vi "waitingStop.vi"(2 "error in (no error)":errorcluster, 3 "UART in":refnum<visa-resource-name>) -> (0 "error out":errorcluster, 1 "UART out":refnum<visa-resource-name>)   [LabVIEW 2016]
panel:
  out "String":string
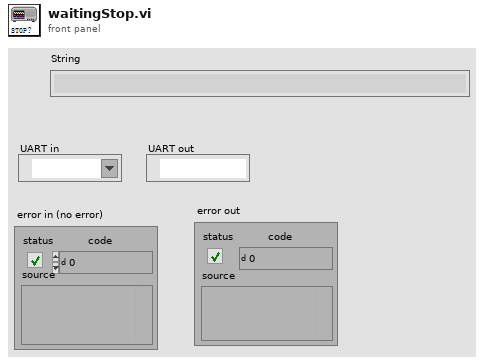
[diagram p1: front panel]
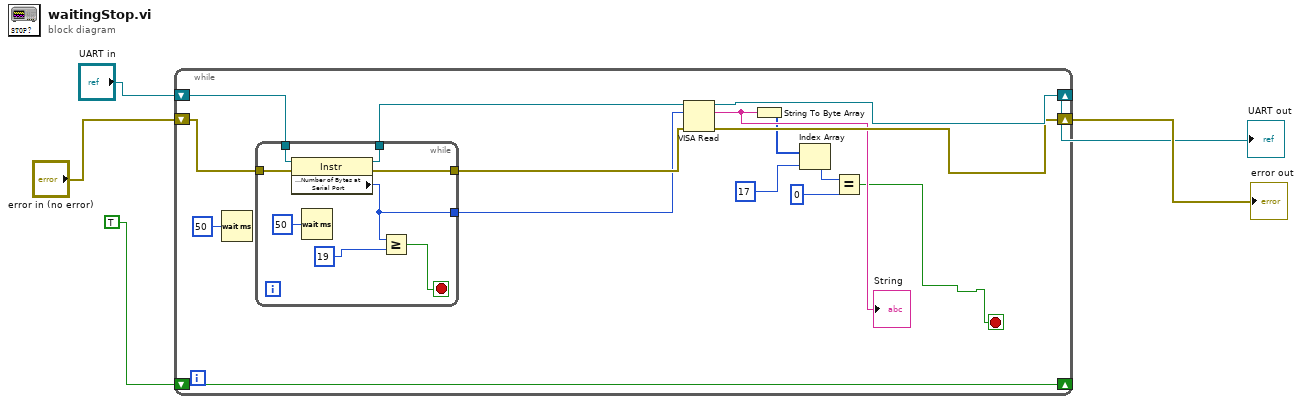
[diagram p0: block diagram]
diagram:
  n1 = while {
    shift-right: [w18] -> w2
    shift-left: "UART in" -> [w10]
    shift-right: [w17] -> w3
    shift-left: "error in (no error)" -> [w11]
    shift-right: [w16] -> _
    shift-left: TRUE -> [w16]
    stop <- w12 stop-if-true
    n2 = Wait (ms)(milliseconds to wait=u32 50) -> ()  [unwired: 1 out]
    n3 = while {
      tunnel: w11 -> [w26]
      tunnel: w10 -> [w25]
      tunnel: [w24] -> w9
      tunnel: [w23] -> w8
      tunnel: [w21] -> w7
      stop <- w27 stop-if-true
      n4 = property class="Instr"(reference=w25, error in=w26) -> (reference out=w24:refnum<visa-resource-name>, error out=w23:errorcluster, "Serial Settings:Number of Bytes at Serial Port"=w21:u32)
      n5 = Wait (ms)(milliseconds to wait=u32 50) -> ()  [unwired: 1 out]
      n6 = Greater Or Equal?(x=w21, y=19) -> (x >= y?=w27:bool)
    }
    n7 = VISA Read(VISA resource name=w9, byte count=w7, error in (no error)=w8) -> (VISA resource name out=w18:refnum<visa-resource-name>, read buffer=w15:string, error out=w17:errorcluster)  [unwired: 1 out]
    "String" <- w15
    n8 = String To Byte Array(string=w15) -> (unsigned byte array=w13:u8[])
    n9 = Index Array(array=w13, index=17) -> (element=w20:u8)
    n10 = Equal?(x=w20, y=0) -> (x = y?=w12:bool)
  }
  "error out" <- w3
  "UART out" <- w2
